vi "SSI_Control.vi"(4 "Tineout":i32=1000, 5 "Write Buffer":string, 6 "Number of bytes":u32=4096, 7 "Remote Mode":u16(ring) items=["USB", "RS232", "GPIB", "Ethernet"], 8 "Error in (no error)":errorcluster caption="error out（no error）", 9 "Control":u16(ring) items=["Write", "Read"], 10 "Connection ID in":refnum<k5>, 11 "VISA resource name":refnum<visa-resource-name>) -> (0 "Error out":errorcluster caption="error out", 1 "Read Buffer":string, 2 "Connection ID out":refnum<k5>, 3 "VISA resource  out":refnum<visa-resource-name>)   [LabVIEW 2011]
uses:
  <vilib>/Instr/_visa.llb/VISA Flush IO Buffer Mask.ctl
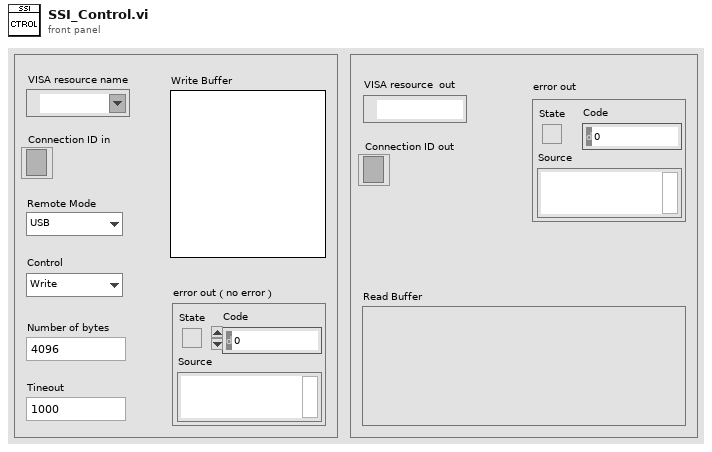
[diagram p1: front panel]
types:
  T1 = enum16{"Standard", "Buffered", "CRLF", "Immediate"}
  T2 = typedef "VISA Flush IO Buffer Mask.ctl" = u16
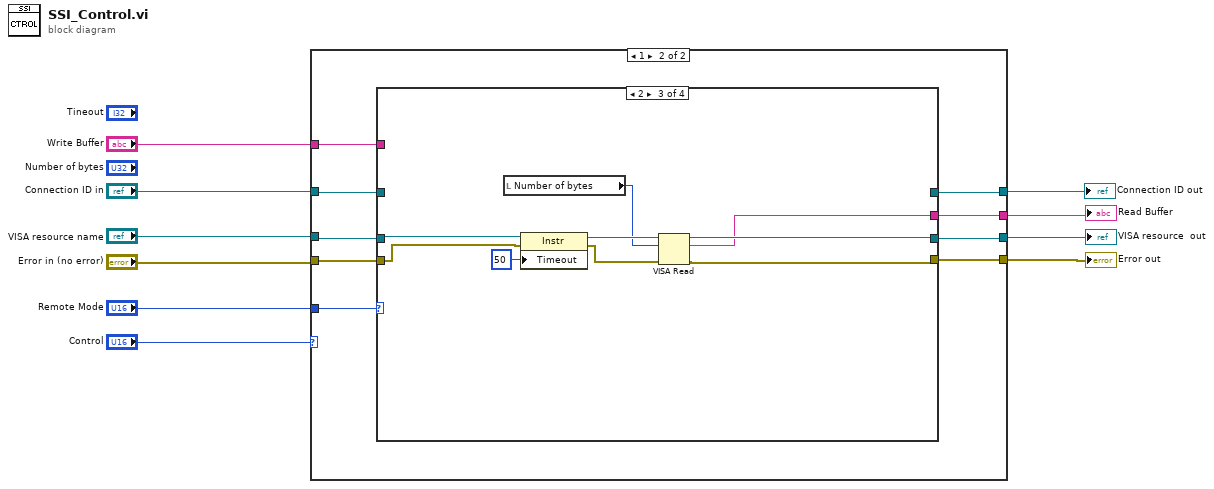
[diagram p0: block diagram]
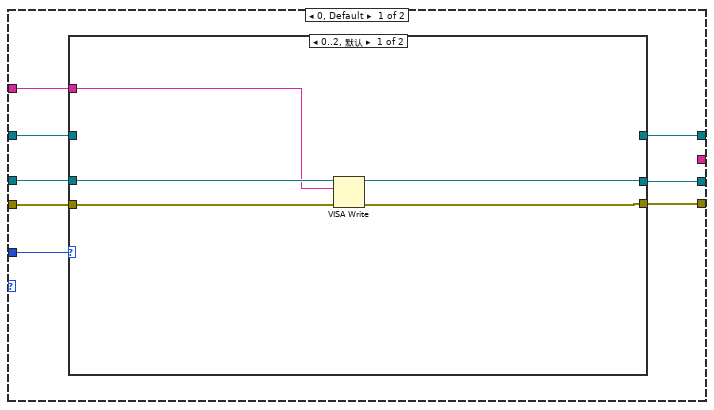
[diagram p2: hidden frame]
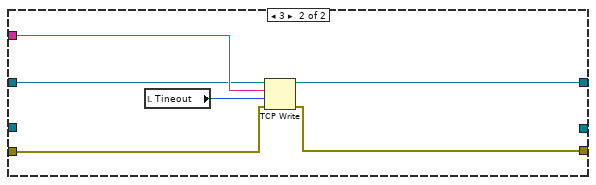
[diagram p3: hidden frame]
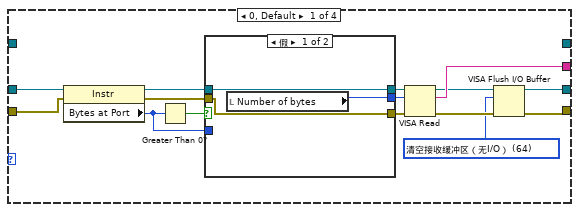
[diagram p4: hidden frame]
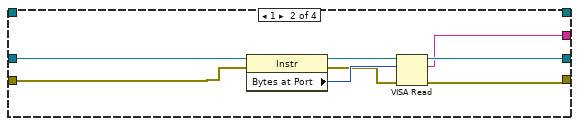
[diagram p6: hidden frame]
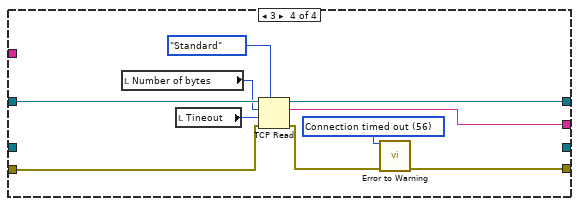
[diagram p7: hidden frame]
diagram:
  n1 = case shown="1" "Control" {
    tunnel: "Remote Mode" -> [w18 w38]
    tunnel: "VISA resource name" -> [w17 w32]
    tunnel: "Error in (no error)" -> [w16 w35]
    tunnel: [w15 w33] -> w3
    tunnel: [w14 w34] -> w1
    tunnel: "Write Buffer" -> [w13 w30]
    tunnel: "Connection ID in" -> [w12 w36]
    tunnel: [w11 w37] -> w5
    tunnel: [_ w31] -> w4
    frame 0, Default {
      n2 = case shown="0..2, 默认" w18 {
        tunnel: w17 -> [w23 _]
        tunnel: w16 -> [w22 w28]
        tunnel: [w20 _] -> w15
        tunnel: [w19 w27] -> w14
        tunnel: w13 -> [w21 w29]
        tunnel: w12 -> [_ w26]
        tunnel: [_ w25] -> w11
        frame 0..2, Default {
          n3 = VISA Write(VISA resource name=w23, write buffer=w21, error in (no error)=w22) -> (VISA resource name out=w20:refnum<visa-resource-name>, error out=w19:errorcluster)  [unwired: 1 out]
        }
        frame 3 {
          n4 = local read "Tineout"() -> (w24:i32)
          n5 = TCP Write(connection ID=w26, data in=w29, error in (no error)=w28, 9:w24) -> (connection ID out=w25:refnum<k5>, error out=w27:errorcluster)  [unwired: 1 out]
        }
      }
    }
    frame 1 {
      n6 = case shown="2" w38 {
        tunnel: [_ _ _ w86] -> w37
        tunnel: w36 -> [_ _ _ w85]
        tunnel: w35 -> [w51 w61 w68 w84]
        tunnel: [w41 w66 w74 w81] -> w34
        tunnel: [w40 w67 w76 _] -> w33
        tunnel: w32 -> [w52 w62 w69 _]
        tunnel: [w53 w60 w75 w80] -> w31
        tunnel: w30 -> [_ _ _ _]
        frame 0, Default {
          w39 = T2 64 items=["清空接收缓冲区"=16, "向设备写入传输缓冲区"=32, "清空接收缓冲区（无I/O）"=64, "清空传输缓冲区"=128] ("Mask")
          n7 = property class="Instr"(reference=w52, error in=w51) -> (reference out=w49:refnum<visa-resource-name>, error out=w48:errorcluster, "Bytes at Port"=w45:u32)
          n8 = Greater Than 0?(x=w45) -> (x > 0?=w50:bool)
          n9 = case shown="假" w50 {
            tunnel: w49 -> [w56 w59]
            tunnel: w48 -> [w55 w58]
            tunnel: [w56 w59] -> w47
            tunnel: [w55 w58] -> w46
            tunnel: w45 -> [_ w57]
            tunnel: [w54 w57] -> w44
            frame False {
              n10 = local read "Number of bytes"() -> (w54:u32)
            }
            frame True {
            }
          }
          n11 = VISA Read(VISA resource name=w47, byte count=w44, error in (no error)=w46) -> (VISA resource name out=w43:refnum<visa-resource-name>, read buffer=w53:string, error out=w42:errorcluster)  [unwired: 1 out]
          n12 = VISA Flush I/O Buffer(VISA resource name=w43, mask (16)=w39, error in (no error)=w42) -> (VISA resource name out=w40:refnum<visa-resource-name>, error out=w41:errorcluster)
        }
        frame 1 {
          n13 = property class="Instr"(reference=w62, error in=w61) -> (reference out=w63:refnum<visa-resource-name>, error out=w64:errorcluster, "Bytes at Port"=w65:u32)
          n14 = VISA Read(VISA resource name=w63, byte count=w65, error in (no error)=w64) -> (VISA resource name out=w67:refnum<visa-resource-name>, read buffer=w60:string, error out=w66:errorcluster)  [unwired: 1 out]
        }
        frame 2 {
          n15 = local read "Number of bytes"() -> (w70:u32)
          n16 = property class="Instr"(reference=w69, error in=w68, "Timeout"=u32 50 ("General Settings:Timeout Value")) -> (reference out=w72:refnum<visa-resource-name>, error out=w71:errorcluster)
          n17 = VISA Read(VISA resource name=w72, byte count=w70, error in (no error)=w71) -> (VISA resource name out=w76:refnum<visa-resource-name>, read buffer=w75:string, error out=w74:errorcluster)  [unwired: 1 out]
        }
        frame 3 {
          w82 = 56 items=["No Error", "Argument Error", "Memory Full", "Out of Zone", "End of File", "File Already Open", "Generic File IO Error", "File Not Found", "File Permission Error", "Disk Full", "Duplicate Path", "Too Many Files Open", "Not Enabled", "Resource File Not Found", "Cannot Add Resource", "Resource Not Found", "Image Not Found", "Image Memory Error", "Pen Does Not Exist", "Config Bad Type", "Config Token Not Found", "Config Parse Error", "Config Memory Error", "Bad External Code Format", "Bad External Code Offset", "External Code Not Present", "Null Window", "Destroy Window Mixup", "Null Menu", "Print Aborted", "Bad Print Record", "Print Driver Error", "Windows Error During Print", "Memory Error During Print", "Print Dialog Error", "Generic Print Error", "Invalid Device Refnum", "Device Not Found", "Device Parameter Error", "Device Unit Error", "Can't Open Device", "Device Call Aborted", "Generic Error", "Cancelled By User", "Object ID Too Low", "Object ID Too High", "Object Not In Heap", "Unknown Heap", "Bad DefProc ID", "DefProc Not In Table", "Message Out Of Range", "Null Method", "Unknown Message", "Manager Call Not Supported", "Bad address", "Connection In progress", "Connection timed out", "Connection is already in progress", "Network attribute not supported", "Network error", "Address in use", "System out of memory", "Connection aborted", "Connection refused", "Connection is not connected", "Connection is already connected", "Connection closed", "Initialize error (interapplication manager)", "Bad occurrence", "Wait on unbound occurrence handler", "Occurrence queue overflow", "Bad path", "Semaphore not signaled", "Unrecognized type (interapplication manager)"] ("1st Error to Convert")
          n18 = local read "Number of bytes"() -> (w79:u32)
          n19 = local read "Tineout"() -> (w78:i32)
          n20 = TCP Read(connection ID=w85, bytes to read=w79, error in (no error)=w84, 7:T1."Standard" ("模式（标准）"), 9:w78) -> (connection ID out=w86:refnum<k5>, data out=w80:string, error out=w83:errorcluster)
          n21 = call <vilib>:"Error to Warning.vi"("1st Error to Convert"=w82, "error in"=w83) -> ("warning out"=w81:errorcluster)  [unwired: 13 in]
        }
      }
    }
  }
  "Connection ID out" <- w5
  "VISA resource  out" <- w3
  "Error out" <- w1
  "Read Buffer" <- w4
